vi "RT Driver VI.vi"(7 "Operation":T1, 11 "Device Reference in":T2 format="%.0x") -> (0 "Error Code":i32)   [LabVIEW 2015, in "Instrument Addon Engine.lvlib"]
uses:
  Instrument Addon Engine.lvlib
  <vilib>/NI Veristand/Custom Device API/Custom Device Item Ref.ctl
  <vilib>/NI Veristand/Custom Device API/Hardware Interface Driver VI Operation.ctl
  SubVIs/Error Handling API/Controls/Error Handling Cluster.ctl
  Types/Commands RT Configuration Cluster.ctl
  Shared/Types/Compiled Settings.ctl
  Shared/Types/Command Parameters.ctl
  Shared/Types/Linked Channel Cluster.ctl
  <vilib>/NI Veristand/Custom Device API/Block Data Reference.ctl
  <vilib>/NI Veristand/Custom Device API/Data Reference.ctl
  Shared/Types/Response RT Configuration Cluster.ctl
  Shared/Types/Response Parameters.ctl
  Shared/Types/Response Wait Type.ctl
  Shared/Types/Message Parameters.ctl
  Shared/Types/Message Generation Type.ctl
  Shared/Types/External Trigger Refs.ctl
  Types/FIFO References.ctl
  Protections.lvlibp/Parent Protection/Protection.lvclass
  Protocols.lvlibp/Protocol Parent/Protocol Parent.lvclass
  <vilib>/NI Veristand/Custom Device API/NI VeriStand - Get Channel Value by Data Reference.vi
  <vilib>/NI Veristand/Custom Device API/NI VeriStand - Set Channel Value by Data Reference.vi
  <vilib>/NI Veristand/Custom Device API/NI VeriStand - Get Channel Values by Block Data Reference.vi
  Shared/Constants.vi
  <vilib>/NI Veristand/Custom Device API/Global Data Refs.vi
  <vilib>/NI Veristand/Custom Device Tools/Custom Device Utility Library/Custom Device Utility Library.lvlib
  SubVIs/Inline Async API/Inline Async API.lvlib
  SubVIs/Error Handling API/Error Handling API.lvlib
  Shared/Instrument Addon Shared.lvlib
  <vilib>/NI Veristand/Custom Device API/Custom Device API.lvlib
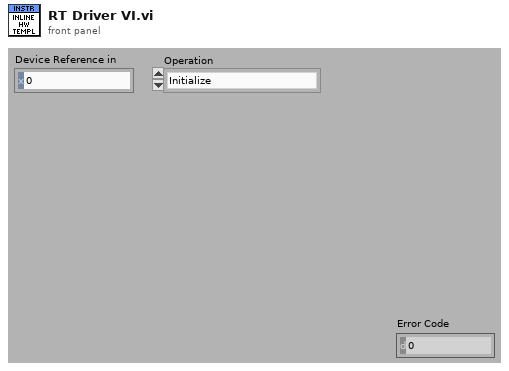
[diagram p1: front panel]
types:
  T1 = typedef "Custom Device API.lvlib/Hardware Interface Driver VI Operation.ctl" = enum16{"Initialize", "Start", "Read Data from HW", "Write Data to HW", "Close"}
  T2 = typedef "Custom Device API.lvlib/Custom Device Item Ref.ctl" = u64
  T3 = typedef "Instrument Addon Engine.lvlib/Error Handling API.lvlib/Error Handling Cluster.ctl" = cluster{"Error Process Q":refnum<queue>, "Process Qs":refnum<queue>[]}
  T4 = typedef "Instrument Addon Engine.lvlib/Commands RT Configuration Cluster.ctl" = cluster{"Compiled":T5, "FIFOs":T16, "Protection Settings":refnum<class "Protection.lvclass">[], "Protocol":refnum<class "Protocol Parent.lvclass">}
  T5 = typedef "Instrument Addon Shared.lvlib/Compiled Settings.ctl" = cluster{"Command Parameters":T6[], "MetaData Lookup":variant, "MetaData":cluster{"Refs":T8[], "Values":dbl[]}, "Triggers":cluster{"Chan Refs":T9[], "Prev. Values":dbl[]}, "Statuses":cluster{"Refs":T9[], "Values":dbl[]}, "Name":string, "Data Lookup":variant, "Response Parameters":T10[], "Data":cluster{"Refs":T9[], "Values":dbl[]}, "Periodic Enable":cluster{"Refs":T8[], "Values":dbl[]}, "Message Generation Settings":T13[], "Wait Value Lookup":variant, "Wait Values":cluster{"Refs":T8[], "Values":dbl[]}, "Decimation":u32, "External Channels":T15}
  T6 = typedef "Instrument Addon Shared.lvlib/Command Parameters.ctl" = cluster{"Command":string, "Linked Channels":T7[], "Pad":bool, "Length":u32, "Pad Value":u8}
  T7 = typedef "Instrument Addon Shared.lvlib/Linked Channel Cluster.ctl" = cluster{"Variable Name":string, "GUID":string}
  T8 = typedef "Custom Device API.lvlib/Block Data Reference.ctl" = cluster{"Data Reference":T9, "Offset":u64, "Length":u64}
  T9 = typedef "Custom Device API.lvlib/Data Reference.ctl" = i32
  T10 = typedef "Instrument Addon Shared.lvlib/Response RT Configuration Cluster.ctl" = cluster{"Reponse Parameters":T11, "Use?":bool}
  T11 = typedef "Instrument Addon Shared.lvlib/Response Parameters.ctl" = cluster{"Response":string, "Linked Channels":T7[], "Type Value":dbl, "Wait Type":T12, "Use Channel":bool, "Channel Path":string}
  T12 = typedef "Instrument Addon Shared.lvlib/Response Wait Type.ctl" = enum16{"Byte Count", "Wait sec"}
  T13 = typedef "Instrument Addon Shared.lvlib/Message Parameters.ctl" = cluster{"Generation Type":T14, "Period":dbl, "Include Protection":bool, "Type":string}
  T14 = typedef "Instrument Addon Shared.lvlib/Message Generation Type.ctl" = enum16{"Trigger Only", "Periodic & Trigger"}
  T15 = typedef "Instrument Addon Shared.lvlib/External Trigger Refs.ctl" = cluster{"Channels":T9[], "Triggers":T9[], "Values":dbl[]}
  T16 = typedef "Instrument Addon Engine.lvlib/FIFO References.ctl" = cluster{"Statuses.Write to VS":refnum<k33>, "MetaData.Read from VS":refnum<k33>, "Trigger.Write to VS":refnum<k33>, "Trigger.Read from VS":refnum<k33>, "Periodic Enable.Read from VS":refnum<k33>, "Data.Write to VS":refnum<k33>, "Wait.Read from VS":refnum<k33>}
  T17 = cluster{"Async VI":refnum<vi>[], "Error Handling Refs":T3, "Error":errorcluster, "Parameters":T4}
  T18 = cluster{"Chan Refs":T9[], "Previous Chan Values":dbl[]}
  T19 = cluster{"Block Data Refs":T8[], "Previous Chan Values":dbl[]}
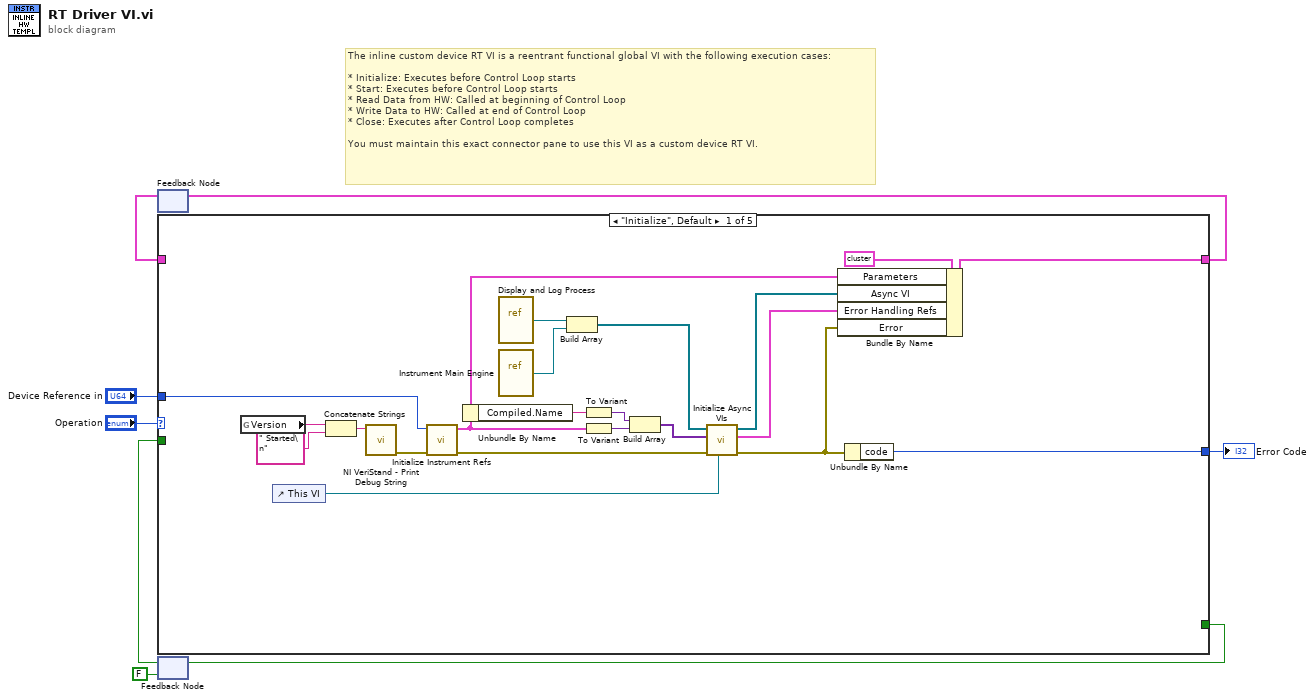
[diagram p0: block diagram]
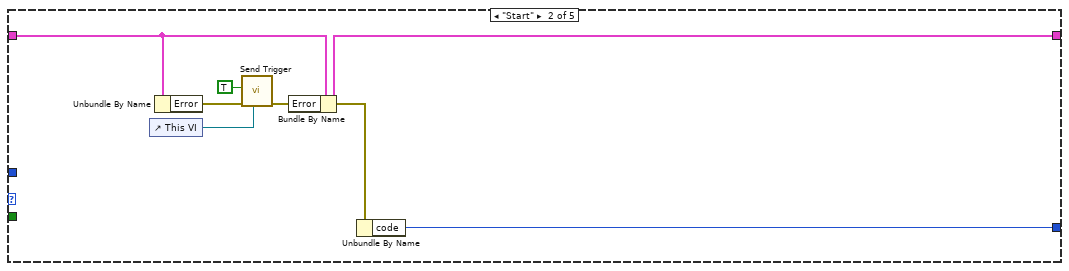
[diagram p2: hidden frame]
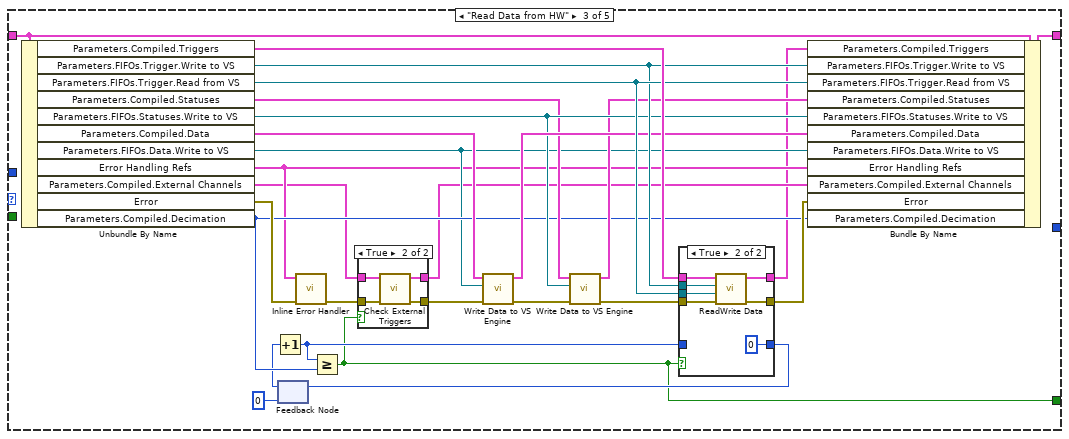
[diagram p3: hidden frame]
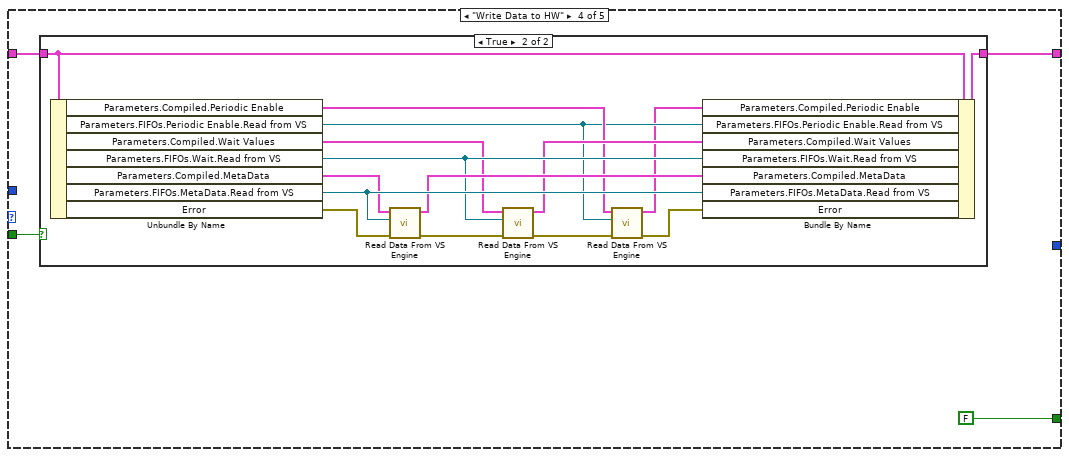
[diagram p6: hidden frame]
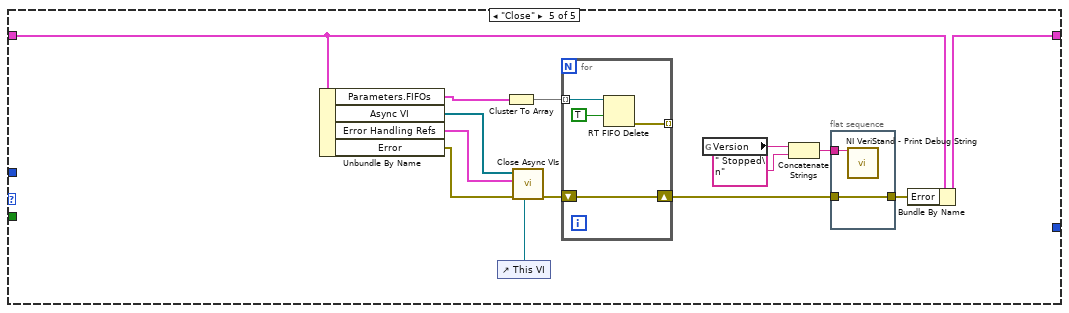
[diagram p8: hidden frame]
diagram:
  # "The inline custom device RT VI is a reentrant functional global VI with the following execution cases:\n\n* Initialize: Executes before Control Loop starts\n* Start: Executes before Control Loop starts\n* Read Data from HW: Called at beginning of Control Loop\n* Write Data to HW: Called at end of Control Loop\n* Close: Executes after Control Loop completes\n\nYou must maintain this exact connector pane to use this VI as a custom device RT VI."
  n1 = feedback #1() -> (w6:T17)  [unwired: 1 out]
  n2 = feedback #2(FALSE) -> (w2:bool)
  n3 = case shown="\"Initialize\", Default" "Operation" {
    tunnel: [w25 w31 w63 w83 w112] -> w7
    tunnel: w6 -> [_ w32 w60 w82 w113]
    tunnel: "Device Reference in" -> [w21 _ _ _ _]
    tunnel: [w29 w36 _ _ _] -> w4
    tunnel: [_ _ w38 FALSE _] -> w3
    tunnel: w2 -> [_ _ _ w81 _]
    frame "Initialize", Default {
      n4 = global read "Constants.vi" "Version"() -> (w23:string)
      n5 = control-ref of="This VI"() -> (w27:refnum<vi>)
      n6 = Concatenate Strings(w23, " Started\n" ("string")) -> (w17:string)
      n7 = call <vilib>:"NI VeriStand - Print Debug String.vi"("Message"=w17) -> ("error out"=w22:errorcluster)  [unwired: 10 in]
      n8 = call "Initialize Instrument Refs.vi"("error in (no error)"=w22, "Device Reference in"=w21) -> ("error out"=w16:errorcluster, "Parameters"=w14:T4)  [unwired: 8 in]
      n9 = Unbundle By Name(w14) -> ("Compiled.Name"=w13:string)
      n10 = vi-ref "Display and Log Process.vi"() -> (w28:refnum<vi>)
      n11 = vi-ref "Instrument Main Engine.vi"() -> (w18:refnum<vi>)
      n12 = Build Array(w28, w18) -> (w10:refnum<vi>[])
      n13 = To Variant(anything=w13) -> (Variant=w12:variant)
      n14 = To Variant(anything=w14) -> (Variant=w20:variant)
      n15 = Build Array(w12, w20) -> (w19:variant[])
      n16 = call "Initialize Async VIs.vi"("VI in"=w27, "error in (no error)"=w16, "Async VI Parameters"=w19, "Async VI Refs"=w10) -> ("error out"=w15:errorcluster, "Error Handling Refs"=w11:T3, "Async VI Refs out"=w9:refnum<vi>[])  [unwired: 5 in]
      n17 = Bundle By Name(cluster=T17 {"Async VI"=[], "Error Handling Refs"={"Error Process Q"=refnum, "Process Qs"=[]}, "Error"={"status"=FALSE, "code"=0, "source"=""}, "Parameters"={"Compiled"={"Command Parameters"=[], "MetaData Lookup"=variant, "MetaData"={"Refs"=[], "Values"=[]}, "Triggers"={"Chan Refs"=[], "Prev. Values"=[]}, "Statuses"={"Refs"=[], "Values"=[]}, "Name"="", "Data Lookup"=variant, "Response Parameters"=[], "Data"={"Refs"=[], "Values"=[]}, "Periodic Enable"={"Refs"=[], "Values"=[]}, "Message Generation Settings"=[], "Wait Value Lookup"=variant, "Wait Values"={"Refs"=[], "Values"=[]}, "Decimation"=0, "External Channels"={"Channels"=[], "Triggers"=[], "Values"=[]}}, "FIFOs"={"Statuses.Write to VS"=refnum, "MetaData.Read from VS"=refnum, "Trigger.Write to VS"=refnum, "Trigger.Read from VS"=refnum, "Periodic Enable.Read from VS"=refnum, "Data.Write to VS"=refnum, "Wait.Read from VS"=refnum}, "Protection Settings"=[], "Protocol"=refnum}}, "Parameters"=w14, "Async VI"=w9, "Error Handling Refs"=w11, "Error"=w15) -> (w25:T17)
      n18 = Unbundle By Name(w15) -> ("code"=w29:i32)
    }
    frame "Start" {
      n19 = control-ref of="This VI"() -> (w34:refnum<vi>)
      n20 = Unbundle By Name(w32) -> ("Error"=w33:errorcluster)
      n21 = call "Send Trigger.vi"("Parent VI"=w34, "error in (no error)"=w33, "notification"=TRUE) -> ("error out"=w30:errorcluster)  [unwired: 8 in]
      n22 = Bundle By Name(cluster=w32, "Error"=w30) -> (w31:T17)
      n23 = Unbundle By Name(w30) -> ("code"=w36:i32)
    }
    frame "Read Data from HW" {
      n24 = Unbundle By Name(w60) -> ("Parameters.Compiled.Triggers"=w61:cluster{"Chan Refs":T9[], "Prev. Values":dbl[]}, "Parameters.FIFOs.Trigger.Write to VS"=w57:refnum<k33>, "Parameters.FIFOs.Trigger.Read from VS"=w58:refnum<k33>, "Parameters.Compiled.Statuses"=w51:cluster{"Refs":T9[], "Values":dbl[]}, "Parameters.FIFOs.Statuses.Write to VS"=w52:refnum<k33>, "Parameters.Compiled.Data"=w56:cluster{"Refs":T9[], "Values":dbl[]}, "Parameters.FIFOs.Data.Write to VS"=w47:refnum<k33>, "Error Handling Refs"=w43:T3, "Parameters.Compiled.External Channels"=w40:T15, "Error"=w62:errorcluster, "Parameters.Compiled.Decimation"=w48:u32)
      n25 = feedback #3(u32 0) -> (w44:u32)
      n26 = Increment(x=w44) -> (x+1=w49:u32)
      n27 = call "Inline Error Handler.vi"("error in"=w62, "Error Handling Cluster"=w43) -> ("error out"=w42:errorcluster)  [unwired: 9 in]
      n28 = Greater Or Equal?(x=w49, y=w48) -> (x >= y?=w38:bool)
      n29 = case shown="True" w38 {
        tunnel: w42 -> [w65 w69]
        tunnel: [w65 w68] -> w41
        tunnel: w40 -> [w64 w67]
        tunnel: [w64 w66] -> w39
        frame False {
        }
        frame True {
          n30 = call "Check External Triggers.vi"("error in (no error)"=w69, "Refs"=w67) -> ("error out"=w68:errorcluster, "Refs"=w66:T15)  [unwired: 8 in]
        }
      }
      n31 = call "Write Data to VS Engine.vi"("error in"=w41, "Write to VS Engine FIFO"=w47, "Channel Pairs"=w56) -> ("error out"=w54:errorcluster, "Channel Pairs Out"=w55:T18)  [unwired: 6 in, 1 out]
      n32 = call "Write Data to VS Engine.vi"("error in"=w54, "Write to VS Engine FIFO"=w52, "Channel Pairs"=w51) -> ("error out"=w53:errorcluster, "Channel Pairs Out"=w50:T18)  [unwired: 6 in, 1 out]
      n33 = case shown="True" w38 {
        tunnel: w61 -> [w70 w79]
        tunnel: [w72 w78] -> w59
        tunnel: w58 -> [_ w77]
        tunnel: w57 -> [_ w76]
        tunnel: [w70 w75] -> w37
        tunnel: w53 -> [w72 w74]
        tunnel: [w71 u32 0] -> w45
        tunnel: w49 -> [w71 _]
        frame False {
        }
        frame True {
          n34 = call "ReadWrite Data.vi"("error in"=w74, "Read from VS Engine FIFO"=w77, "Write to VS Engine FIFO"=w76, "Channel Pairs"=w79) -> ("error out"=w78:errorcluster, "Channel Pairs Out"=w75:T18)  [unwired: 5 in, 1 out]
        }
      }
      n35 = feedback-in #3(w45) -> ()
      n36 = Bundle By Name(cluster=w60, "Parameters.Compiled.Triggers"=w37, "Parameters.FIFOs.Trigger.Write to VS"=w57, "Parameters.FIFOs.Trigger.Read from VS"=w58, "Parameters.Compiled.Statuses"=w50, "Parameters.FIFOs.Statuses.Write to VS"=w52, "Parameters.Compiled.Data"=w55, "Parameters.FIFOs.Data.Write to VS"=w47, "Error Handling Refs"=w43, "Parameters.Compiled.External Channels"=w39, "Error"=w59, "Parameters.Compiled.Decimation"=w48) -> (w63:T17)
    }
    frame "Write Data to HW" {
      n37 = case shown="True" w81 {
        tunnel: [w84 w99] -> w83
        tunnel: w82 -> [w84 w98]
        frame False {
        }
        frame True {
          n38 = Unbundle By Name(w98) -> ("Parameters.Compiled.Periodic Enable"=w87:cluster{"Refs":T8[], "Values":dbl[]}, "Parameters.FIFOs.Periodic Enable.Read from VS"=w86:refnum<k33>, "Parameters.Compiled.Wait Values"=w89:cluster{"Refs":T8[], "Values":dbl[]}, "Parameters.FIFOs.Wait.Read from VS"=w90:refnum<k33>, "Parameters.Compiled.MetaData"=w95:cluster{"Refs":T8[], "Values":dbl[]}, "Parameters.FIFOs.MetaData.Read from VS"=w97:refnum<k33>, "Error"=w96:errorcluster)
          n39 = call "Read Data From VS Engine.vi"("error in"=w96, "Read from VS Engine FIFO"=w97, "Channel Pairs"=w95) -> ("error out"=w93:errorcluster, "Channel Pairs"=w94:T19)  [unwired: 6 in, 1 out]
          n40 = call "Read Data From VS Engine.vi"("error in"=w93, "Read from VS Engine FIFO"=w90, "Channel Pairs"=w89) -> ("error out"=w92:errorcluster, "Channel Pairs"=w88:T19)  [unwired: 6 in, 1 out]
          n41 = call "Read Data From VS Engine.vi"("error in"=w92, "Read from VS Engine FIFO"=w86, "Channel Pairs"=w87) -> ("error out"=w91:errorcluster, "Channel Pairs"=w85:T19)  [unwired: 6 in, 1 out]
          n42 = Bundle By Name(cluster=w98, "Parameters.Compiled.Periodic Enable"=w85, "Parameters.FIFOs.Periodic Enable.Read from VS"=w86, "Parameters.Compiled.Wait Values"=w88, "Parameters.FIFOs.Wait.Read from VS"=w90, "Parameters.Compiled.MetaData"=w94, "Parameters.FIFOs.MetaData.Read from VS"=w97, "Error"=w91) -> (w99:T17)
        }
      }
    }
    frame "Close" {
      n43 = Unbundle By Name(w113) -> ("Parameters.FIFOs"=w106:T16, "Async VI"=w105:refnum<vi>[], "Error Handling Refs"=w104:T3, "Error"=w103:errorcluster)
      n44 = control-ref of="This VI"() -> (w111:refnum<vi>)
      n45 = Cluster To Array(cluster=w106) -> (array=w100:refnum<k33>[])
      n46 = call "Close Async VIs.vi"("TopLevel VI"=w111, "error in (no error)"=w103, "Error Handling Refs"=w104, "Async VI"=w105) -> ("error out"=w102:errorcluster)  [unwired: 7 in]
      n47 = for {
        tunnel: w100 -> [w117] mode=indexing
        tunnel: [w116] -> _ mode=indexing
        shift-right: [w114] -> w101
        shift-left: w102 -> [w114]
        n48 = RT FIFO Delete(0:w117, 2:TRUE ("force destroy? (F)")) -> (11:w116:errorcluster)  [unwired: 1 in]
      }
      n49 = global read "Constants.vi" "Version"() -> (w107:string)
      n50 = Concatenate Strings(w107, " Stopped\n" ("string")) -> (w108:string)
      n51 = flat-sequence {
        tunnel: [w119] -> w109
        tunnel: w101 -> [w119]
        tunnel: w108 -> [w118]
        frame #0 {
          n52 = call <vilib>:"NI VeriStand - Print Debug String.vi"("Message"=w118) -> ()  [unwired: 10 in, 1 out]
        }
      }
      n53 = Bundle By Name(cluster=w113, "Error"=w109) -> (w112:T17)
    }
  }
  "Error Code" <- w4
  n54 = feedback-in #1(w7) -> ()
  n55 = feedback-in #2(w3) -> ()
